vi "模拟输入_电流_连续.vi"() -> ()   [LabVIEW 2013]
doc: "This example demonstrates how to acquire a continuous data."
uses:
  <userlib>/ArtDAQ/_SubVI/ArtDAQ_CreateAICurrentChan.vi
  <userlib>/ArtDAQ/_SubVI/ArtDAQ_CfgSampClkTiming.vi
  <userlib>/ArtDAQ/_SubVI/ArtDAQ_CfgDigEdgeStartTrig.vi
  <userlib>/ArtDAQ/_SubVI/ArtDAQ_CfgAnlgEdgeStartTrig.vi
  <userlib>/ArtDAQ/_SubVI/ArtDAQ_CfgAnlgWindowStartTrig.vi
  <userlib>/ArtDAQ/_SubVI/ArtDAQ_Read Analog DBL NChan NSamp.vi
panel:
  in  "外部分流电阻值(Ω)":dbl=249.0 format="%.2f"
  in  "分流电阻位置":i32(ring)=-1 items=["默认"=-1, "内部"=10200, "外部"=10167]
  in  "触发模式":enum32{"无触发", "数字边沿", "模拟边沿", "模拟窗"}(tab)
  in  "触发源":string="/Dev1/PFI1"
  in  "触发边沿":i32(ring)=10280 items=["上升"=10280, "下降"=10171]
  in  "触发电平(V)":dbl
  in  "触发源":string(combo)="Dev1/ai0"
  in  "斜率":i32(ring)=10280 items=["上升"=10280, "下降"=10171]
  in  "触发条件":i32(ring)=10163 items=["进入窗"=10163, "离开窗"=10208]
  in  "窗顶部":dbl=0.5
  in  "窗底部":dbl
  in  "触发源":string(combo)="Dev1/ai0"
  in  "停止":bool
  out "Waveform":dbl[][](graph)
  in  "采样频率":dbl=10000.0 format="%#_13g"
  in  "每通道采样点数":i32=1000
  in  "最小电流(A)":dbl format="%#_13g"
  in  "最大电流(A)":dbl=0.02 format="%#_13g"
  in  "物理通道":string(combo)="Dev1/ai0"
  out "错误":errorcluster
  # "通道属性"
  # "定时"
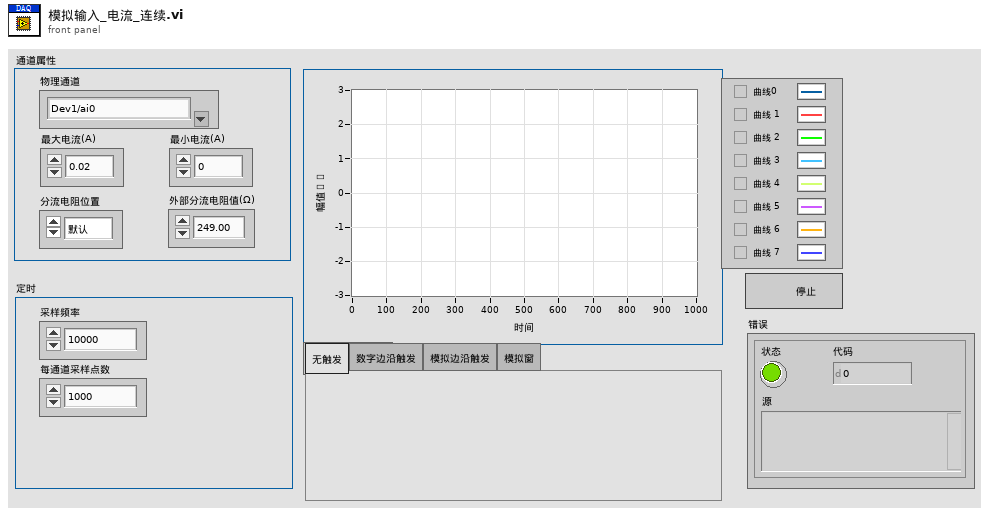
[diagram p1: front panel]
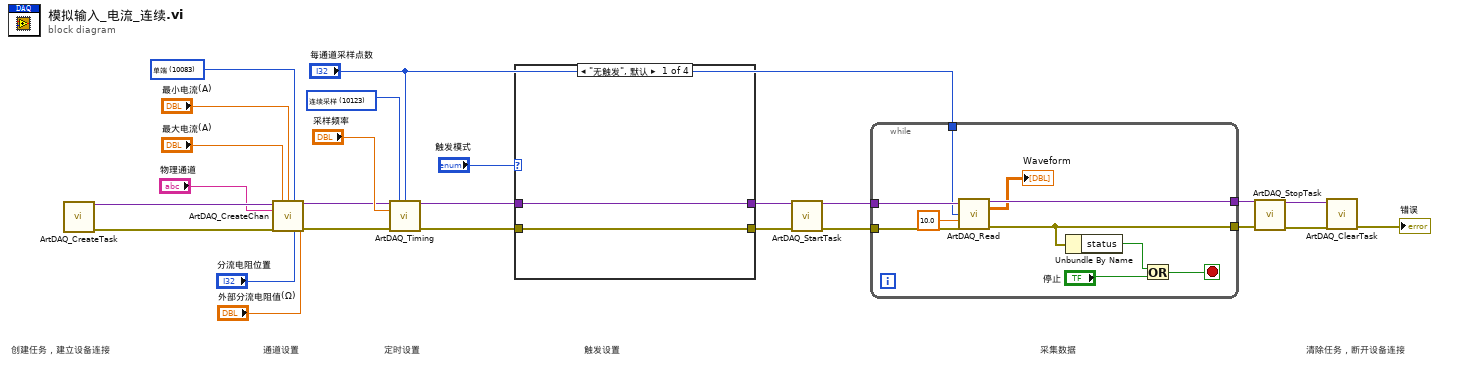
[diagram p0: block diagram]
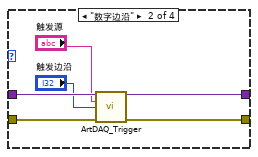
[diagram p2: hidden frame]
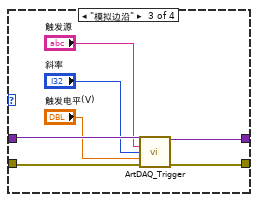
[diagram p3: hidden frame]
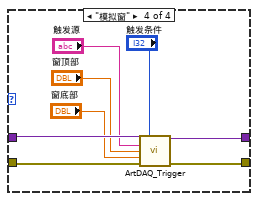
[diagram p4: hidden frame]
diagram:
  w22 = 10083 items=["默认"=-1, "单端"=10083, "非参考单端"=10078, "差分"=10106, "伪差分"=12529] ("接地方式")
  w3 = 10123 items=["有限点采样"=10178, "连续采样"=10123] ("SampleMode")
  # "清除任务，断开设备连接"
  # "采集数据"
  # "触发设置"
  # "定时设置"
  # "通道设置"
  # "创建任务，建立设备连接"
  n1 = call <userlib>:"ArtDAQ_CreateTask.vi"() -> ("任务句柄"=w15:variant, "错误输出"=w25:errorcluster)  [unwired: 14 in]
  n2 = call-poly <userlib>:"ArtDAQ_CreateChan.vi"("任务句柄"=w15, "最大值"="最大电流(A)", "最小值"="最小电流(A)", "接线端配置"=w22, "物理通道"="物理通道", "外部分流电阻值"="外部分流电阻值(Ω)", "错误输入"=w25, "分流电阻位置"="分流电阻位置") -> ("任务句柄"=w4:variant, "错误输出"=w21:errorcluster)  [unwired: 6 in]
  n3 = call-poly <userlib>:"ArtDAQ_Timing.vi"("任务句柄"=w4, "采样模式"=w3, "每通道采样数"="每通道采样点数", "采样率"="采样频率", "错误输入"=w21) -> ("任务句柄"=w9:variant, "错误输出"=w7:errorcluster)  [unwired: 9 in]
  n4 = case shown="\"无触发\", 默认" "触发模式" {
    tunnel: w9 -> [w27 w33 w40 w48]
    tunnel: [w27 w32 w39 w47] -> w8
    tunnel: w7 -> [w26 w30 w37 w45]
    tunnel: [w26 w31 w38 w46] -> w6
    frame "无触发", Default {
    }
    frame "数字边沿" {
      n5 = call-poly <userlib>:"ArtDAQ_Trigger.vi"("任务句柄"=w33, "触发源"="触发源", "边沿"="触发边沿", "错误输入"=w30) -> ("任务句柄"=w32:variant, "错误输出"=w31:errorcluster)  [unwired: 10 in]
    }
    frame "模拟边沿" {
      n6 = call-poly <userlib>:"ArtDAQ_Trigger.vi"("任务句柄"=w40, "触发源"="触发源", "斜率"="斜率", "触发电平"="触发电平(V)", "错误输入"=w37) -> ("任务句柄"=w39:variant, "错误输出"=w38:errorcluster)  [unwired: 9 in]
    }
    frame "模拟窗" {
      n7 = call-poly <userlib>:"ArtDAQ_Trigger.vi"("任务句柄"=w48, "触发条件"="触发条件", "触发源"="触发源", "窗顶部"="窗顶部", "窗底部"="窗底部", "错误输入"=w45) -> ("任务句柄"=w47:variant, "错误输出"=w46:errorcluster)  [unwired: 8 in]
    }
  }
  n8 = call <userlib>:"ArtDAQ_StartTask.vi"("任务句柄"=w8, "错误输入"=w6) -> ("任务句柄"=w18:variant, "错误输出"=w17:errorcluster)  [unwired: 12 in]
  n9 = while {
    tunnel: w18 -> [w58]
    tunnel: w17 -> [w57]
    tunnel: "每通道采样点数" -> [w56]
    tunnel: [w54] -> w14
    tunnel: [w53] -> w13
    stop <- w51 stop-if-true
    n10 = call-poly <userlib>:"ArtDAQ_Read.vi"("任务句柄"=w58, "每通道采样数"=w56, "超时s"=10.0 ("Timeout"), "错误输入"=w57) -> ("任务句柄"=w54:variant, "数据"=→"Waveform":dbl[][], "错误输出"=w53:errorcluster)  [unwired: 8 in, 1 out]
    n11 = Unbundle By Name(w53) -> ("status"=w52:bool)
    n12 = Or(x=w52, y="停止") -> (x .or. y?=w51:bool)
  }
  n13 = call <userlib>:"ArtDAQ_StopTask.vi"("任务句柄"=w14, "错误输入"=w13) -> ("任务句柄"=w12:variant, "错误输出"=w11:errorcluster)  [unwired: 12 in]
  n14 = call <userlib>:"ArtDAQ_ClearTask.vi"("任务句柄"=w12, "错误输入"=w11) -> ("错误输出"=→"错误":errorcluster)  [unwired: 13 in]
